vi "Scanner Message Loop.vi"(8 "error in (no error)":errorcluster) -> (0 "error out":errorcluster)   [LabVIEW 2020, in "Hiden Scanner.lvlib"]
doc: "Message loop for handling messages pertaining to the acquisition of data from the hardware."
uses:
  Hiden Scanner.lvlib
  support/PCT FGV CMD.ctl
  Acquisition State.ctl
  Scanner Hardware Configuration.ctl
  support/Message Queue/Message Cluster.ctl
  support/Message Queue/Enqueue Message (Single).vi
  <vilib>/Utility/error.llb/Error Cluster From Error Code.vi
  <vilib>/ErrorRing/Error Ring.xnode
  support/Message Queue/Message Queue.lvlib
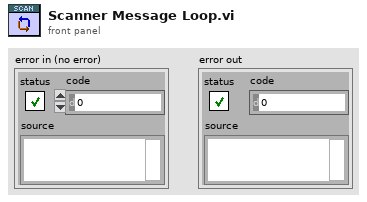
[diagram p1: front panel]
types:
  T1 = typedef "PCT FGV CMD.ctl" = enum16{"INIT", "GET", "SET"}
  T2 = typedef "Message Queue.lvlib/All Message Queues.ctl" = cluster{"UI":refnum<queue>, "Logging":refnum<queue>, "LOG":refnum<queue>, "ALARM":refnum<queue>, "Test":refnum<queue>, "Answer":refnum<queue>, "PLC":refnum<queue>, "DB":refnum<queue>, "Report":refnum<queue>, "OPC":refnum<queue>, "Procedure":refnum<queue>, "PalmSens":refnum<queue>, "SYS 7000 Reader":refnum<queue>, "SWITCH":refnum<queue>, "MOTOR":refnum<queue>, "MOTION":refnum<queue>, "HIDEN":refnum<queue>, "VALVE":refnum<queue>, "MFC":refnum<queue>, "PUMP IN":refnum<queue>, "PUMP OUT":refnum<queue>}
  T3 = typedef "PCT Data REFs.ctl" = cluster{"PLC AI Notifier":refnum<notifier>, "PS Data Queue":refnum<queue>, "BTN Queue":refnum<queue>, "PLC DI notifier":refnum<notifier>, "Timer notifier":refnum<notifier>, "DMM PS":refnum<notifier>, "DMM Gages":refnum<notifier>, "XYZ notifier":refnum<notifier>, "Test Notifier":refnum<notifier>, "Scanner notifier":refnum<notifier>, "OPC Notifier":refnum<notifier>, "HIDEN queue":refnum<queue>}
  T4 = typedef "Hiden Scanner.lvlib/Scanner Hardware Configuration.ctl" = cluster{"Link":cluster{"Connection":enum16{"Serial", "TCP/IP", "USB"}, "Host or IP address (TCP/IP)":string, "Port (Serial/USB)":string}, "VISA resource":refnum<visa-resource-name>, "Writer Queue":refnum<queue>, "Status":bool}
  T5 = typedef "Message Queue.lvlib/Message Cluster.ctl" = cluster{"Message":string, "Message Data":variant}
  T6 = typedef "Hiden Scanner.lvlib/Acquisition State.ctl" = enum16{"Idle", "Initialized"}
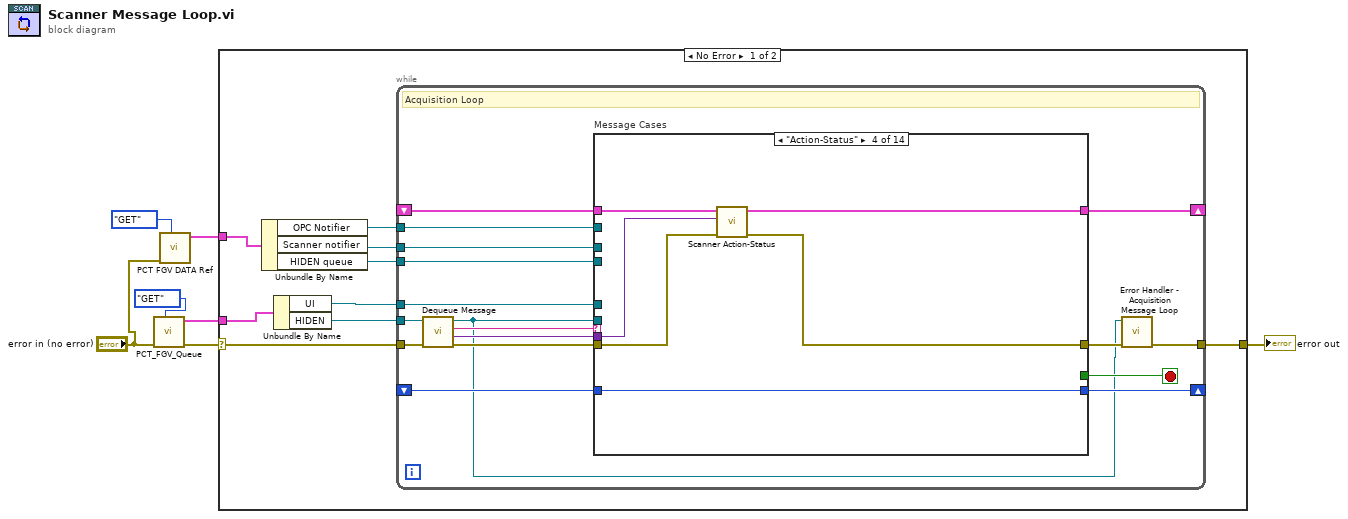
[diagram p0: block diagram]
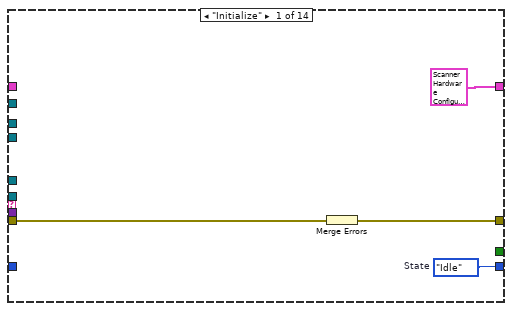
[diagram p2: hidden frame]
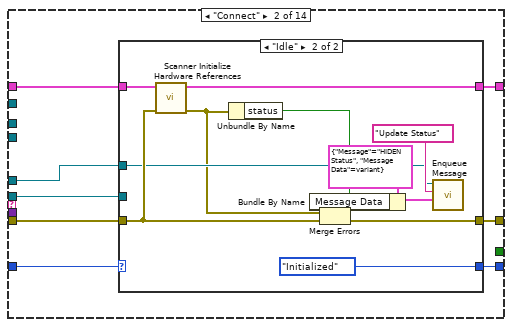
[diagram p3: hidden frame]
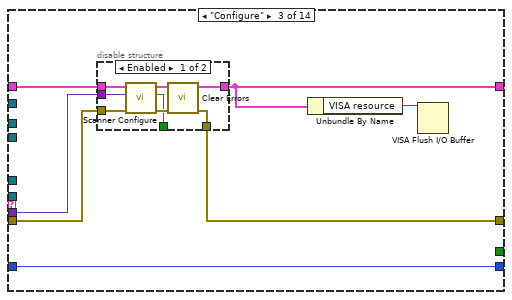
[diagram p5: hidden frame]
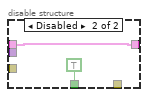
[diagram p6: hidden frame]
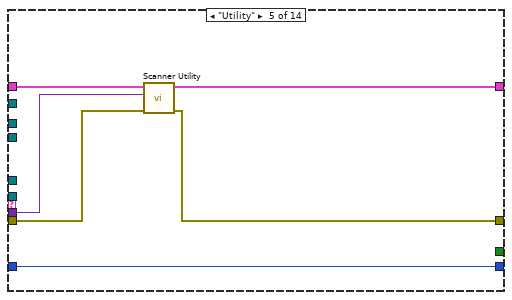
[diagram p7: hidden frame]
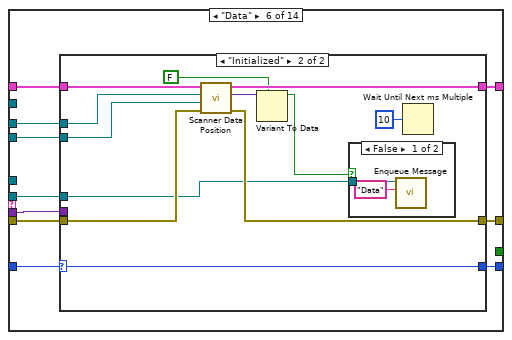
[diagram p8: hidden frame]
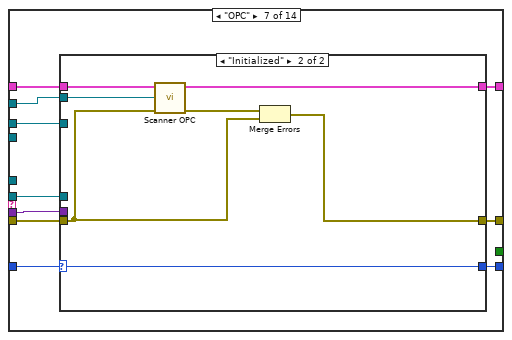
[diagram p11: hidden frame]
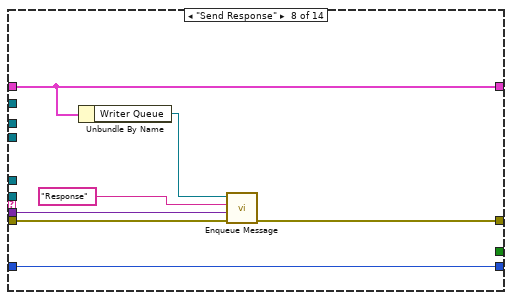
[diagram p13: hidden frame]
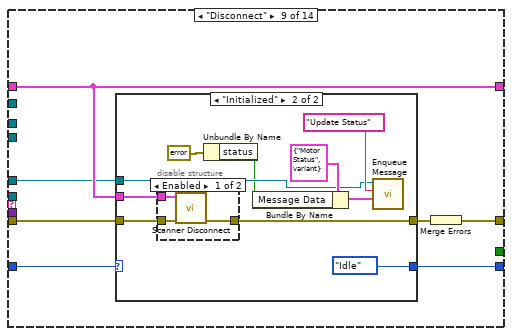
[diagram p14: hidden frame]
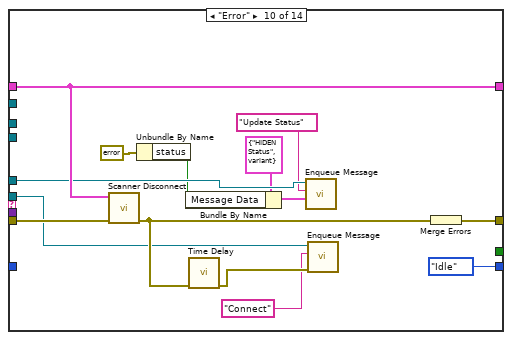
[diagram p17: hidden frame]
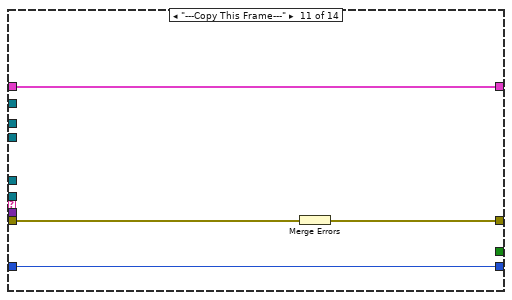
[diagram p18: hidden frame]
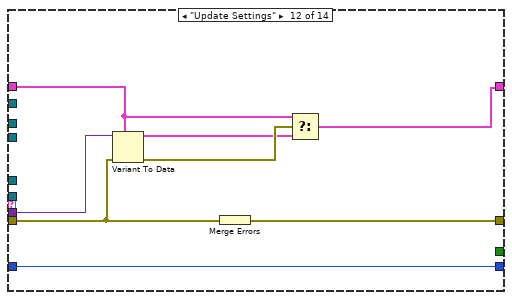
[diagram p19: hidden frame]
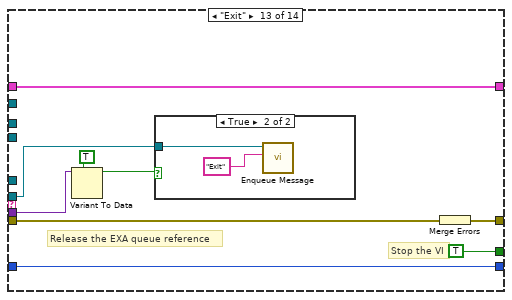
[diagram p20: hidden frame]
diagram:
  n1 = call "PCT_FGV_Queue.vi"("CMD"=PCT_FGV_CMD."GET", "error in (no error)"="error in (no error)") -> ("error out"=w5:errorcluster, "Message Queues out"=w4:T2)  [unwired: 8 in]
  n2 = call "PCT FGV DATA Ref.vi"("CMD"=PCT_FGV_CMD."GET", "error in (no error)"="error in (no error)") -> ("Data REF"=w1:T3)  [unwired: 8 in, 1 out]
  n3 = case shown="No Error" w5 {
    selector: w5 -> [w13 w212]
    tunnel: w4 -> [w16 _]
    tunnel: [w14 w212] -> w7
    tunnel: w1 -> [w11 _]
    frame No Error {
      n4 = Unbundle By Name(w11) -> ("OPC Notifier"=w9:refnum<notifier>, "Scanner notifier"=w10:refnum<notifier>, "HIDEN queue"=w8:refnum<queue>)
      n5 = Unbundle By Name(w16) -> ("UI"=w12:refnum<queue>, "HIDEN"=w15:refnum<queue>)
      n6 = while {
        tunnel: w15 -> [w27]
        shift-right: [w32] -> _
        shift-left: _ -> [w33]
        tunnel: w12 -> [w22]
        shift-right: [w25] -> _
        shift-left: _ -> [w26]
        tunnel: w13 -> [w30]
        tunnel: [w24] -> w14
        tunnel: w10 -> [w20]
        tunnel: w9 -> [w19]
        tunnel: w8 -> [w17]
        stop <- w31 stop-if-true
        # "Acquisition Loop"
        n7 = call "Dequeue Message.vi"("error in (no error)"=w30, "Message Queue"=w27) -> ("error out"=w29:errorcluster, "Message Data"=w28:variant, "Message"=w21:string, "dup Message Queue"=w18:refnum<queue>)  [unwired: 6 in]
        n8 = case "Message Cases" shown="\"Action-Status\"" w21 {
          selector: w21 -> [_ _ _ _ _ _ _ _ _ _ _ _ _ w201]
          tunnel: w18 -> [_ w42 _ _ _ w96 w123 _ _ w165 _ _ w192 _]
          tunnel: w29 -> [w36 w43 w63 w77 w84 w95 w122 w139 w147 w176 w181 w183 w191 _]
          tunnel: [w37 w45 w62 w76 w82 w97 w124 w138 w148 w177 w179 w189 w197 w202] -> w23
          tunnel: w33 -> [_ w44 w64 w78 w86 w93 w120 w136 w145 w175 w180 w185 w196 w204]
          tunnel: [T4 {"Link"={"Connection"=enum."Serial", "Host or IP address (TCP/IP)"="", "Port (Serial/USB)"="COM1"}, "VISA resource"="", "Writer Queue"=refnum, "Status"=FALSE} ("Data Cluster") w41 w61 w79 w83 w94 w121 w136 w145 w175 w180 w184 w196 w204] -> w32
          tunnel: [_ _ _ _ _ _ _ _ _ _ _ _ TRUE _] -> w31
          tunnel: w28 -> [_ _ w65 w80 w85 w90 w117 w137 _ _ _ w188 w190 _]
          tunnel: w22 -> [_ w38 _ _ _ _ _ _ w142 w173 _ _ _ _]
          tunnel: w26 -> [_ w39 w66 w81 w87 w91 w118 w140 w144 _ w178 w182 w195 w203]
          tunnel: [w35 w40 w66 w81 w87 w92 w119 w140 w143 Acquisition_State."Idle" ("State") w178 w182 w195 w203] -> w25
          tunnel: w20 -> [_ _ _ _ _ w89 w116 _ _ _ _ _ _ _]
          tunnel: w19 -> [_ _ _ _ _ _ w115 _ _ _ _ _ _ _]
          tunnel: w17 -> [_ _ _ _ _ w88 _ _ _ _ _ _ _ _]
          frame "Initialize" {
            w35 = Acquisition_State."Idle"  # State
            # "Initialize  - Initialize is currently a no-op.  The hardware initialization takes place in the 'Start' message."
            n9 = Merge Errors(w36) -> (w37:errorcluster)
          }
          frame "Connect" {
            # "Start - Configure and start the acquisition."
            n10 = case shown="\"Idle\"" w39 {
              selector: w39 -> [w46 _]
              tunnel: [w47 w59] -> w45
              tunnel: w44 -> [w48 w58]
              tunnel: w43 -> [w47 w55]
              tunnel: w42 -> [_ _]
              tunnel: [w48 w57] -> w41
              tunnel: [w46 Acquisition_State."Initialized" ("Acquisition State")] -> w40
              tunnel: w38 -> [_ w51]
              frame "Initialized" {
                # "The system is already acquiring. Ignore the \"Start\" message."
              }
              frame "Idle" {
                # "If the system is idle, start the acquisition."
                n11 = call "Scanner Initialize Hardware References.vi"("error in (no error)"=w55, "Hardware Resources in"=w58) -> ("error out"=w49:errorcluster, "Hardware Resources out"=w57:T4)  [unwired: 8 in]
                n12 = Unbundle By Name(w49) -> ("status"=w50:bool)
                n13 = Bundle By Name(cluster=T5 {"Message"="HIDEN Status", "Message Data"=variant} ("Message Cluster"), "Message Data"=w50) -> (w53:T5)
                n14 = Merge Errors(w49, w55) -> (w59:errorcluster)
                n15 = call-poly "Enqueue Message.vi"("Message Data"=w53, "Message"="Update Status", "Message Queue"=w51) -> ()  [unwired: 7 in, 2 out]
              }
            }
          }
          frame "Configure" {
            # "Start - Configure and start the acquisition."
            n16 = disable-structure shown="Enabled" {
              disable-tunnel: w65 -> [w73 _]
              disable-tunnel: w64 -> [w72 w75]
              disable-tunnel: w63 -> [w71 _]
              disable-tunnel: [w69 w75] -> w61
              disable-tunnel: [w68 _] -> w62
              disable-tunnel: [w67 TRUE ("Send Resp")] -> _
              frame Enabled {
                n17 = call "Scanner Configure.vi"("error in (no error)"=w71, "Message Data"=w73, "Data Cluster"=w72) -> ("error out"=w70:errorcluster, "Send Resp"=w67:bool, "Data Cluster out"=w69:T4)  [unwired: 6 in]
                n18 = call <vilib>:"Clear Errors.vi"("error in (no error)"=w70) -> ("error out"=w68:errorcluster)  [unwired: 5 in, 1 out]
              }
              frame Disabled {
              }
            }
            n19 = Unbundle By Name(w61) -> ("VISA resource"=w60:refnum<visa-resource-name>)
            n20 = VISA Flush I/O Buffer(VISA resource name=w60) -> ()  [unwired: 2 in, 2 out]
          }
          frame "Action-Status" {
            # "Start - Configure and start the acquisition."
            n21 = call "Scanner Action-Status.vi"("error in (no error)"=w77, "Message Data"=w80, "Data Cluster"=w78) -> ("error out"=w76:errorcluster, "Data Cluster out"=w79:T4)  [unwired: 7 in]
          }
          frame "Utility" {
            # "Start - Configure and start the acquisition."
            n22 = call "Scanner Utility.vi"("error in (no error)"=w84, "Message Data"=w85, "Data Cluster"=w86) -> ("error out"=w82:errorcluster, "Data Cluster out"=w83:T4)  [unwired: 7 in]
          }
          frame "Data" {
            # "Acquire - Acquire data from the hardware. Since this is a continuous acquisition, this message will always message itself to run again."
            n23 = case shown="\"Initialized\"" w91 {
              selector: w91 -> [w98 w112]
              tunnel: [w99 w109] -> w97
              tunnel: w96 -> [_ w106]
              tunnel: w95 -> [w99 w108]
              tunnel: [w100 w110] -> w94
              tunnel: w93 -> [w100 w111]
              tunnel: [w98 w112] -> w92
              tunnel: w90 -> [_ _]
              tunnel: w89 -> [_ w107]
              tunnel: w88 -> [_ w101]
              frame "Idle" {
              }
              frame "Initialized" {
                # "Read  data"
                n24 = call "Scanner Data Position.vi"("error in (no error)"=w108, "queue"=w101, "Scanner notifier"=w107, "Hardware Resources in"=w111) -> ("error out"=w109:errorcluster, "Message Data Out"=w104:variant, "Hardware Resources out"=w110:T4)  [unwired: 5 in]
                n25 = Variant To Data(type=FALSE, Variant=w104) -> (data=w102:bool)  [unwired: 1 in, 1 out]
                n26 = case shown="False" w102 {
                  tunnel: w106 -> [w114 _]
                  frame False {
                    n27 = call-poly "Enqueue Message.vi"("Message"="Data", "Message Queue"=w114) -> ()  [unwired: 8 in, 2 out]
                  }
                  frame True {
                  }
                }
                n28 = Wait Until Next ms Multiple(millisecond multiple=u32 10) -> ()  [unwired: 1 out]
              }
            }
          }
          frame "OPC" {
            # "Acquire - Acquire data from the hardware. Since this is a continuous acquisition, this message will always message itself to run again."
            n29 = case shown="\"Initialized\"" w118 {
              selector: w118 -> [w125 w133]
              tunnel: [w126 w134] -> w124
              tunnel: w123 -> [_ _]
              tunnel: w122 -> [w126 w130]
              tunnel: [w127 w131] -> w121
              tunnel: w120 -> [w127 w132]
              tunnel: [w125 w133] -> w119
              tunnel: w117 -> [_ _]
              tunnel: w116 -> [_ _]
              tunnel: w115 -> [_ w128]
              frame "Idle" {
              }
              frame "Initialized" {
                # "Read  data"
                n30 = call "Scanner OPC.vi"("error in (no error)"=w130, "OPC Notifier"=w128, "Hardware Resources in"=w132) -> ("error out"=w129:errorcluster, "Hardware Resources out"=w131:T4)  [unwired: 7 in]
                n31 = Merge Errors(w129, w130) -> (w134:errorcluster)
              }
            }
          }
          frame "Send Response" {
            # "Acquire - Acquire data from the hardware. Since this is a continuous acquisition, this message will always message itself to run again."
            n32 = Unbundle By Name(w136) -> ("Writer Queue"=w135:refnum<queue>)
            n33 = call-poly "Enqueue Message.vi"("error in (no error)"=w139, "Message Data"=w137, "Message"="Response", "Message Queue"=w135) -> ("error out"=w138:errorcluster)  [unwired: 6 in, 1 out]
          }
          frame "Disconnect" {
            # "Stop - Stop the Acquisition."
            n34 = case shown="\"Initialized\"" w144 {
              selector: w144 -> [w149 _]
              tunnel: w147 -> [w150 w160]
              tunnel: [w150 w159] -> w146
              tunnel: w145 -> [_ w158]
              tunnel: [w149 Acquisition_State."Idle" ("State")] -> w143
              tunnel: w142 -> [_ w152]
              frame "Idle" {
                # "The system is already idle. Ignore the \"Stop\" message."
              }
              frame "Initialized" {
                # "If the system is acquiring, stop the acquisition."
                n35 = disable-structure shown="Enabled" {
                  disable-tunnel: w160 -> [w163 _]
                  disable-tunnel: [w162 _] -> w159
                  disable-tunnel: w158 -> [w161 _]
                  frame Enabled {
                    n36 = call "Scanner Disconnect.vi"("error in (no error)"=w163, "Hardware Resources in"=w161) -> ("error out"=w162:errorcluster)  [unwired: 9 in]
                  }
                  frame Disabled {
                  }
                }
                n37 = Unbundle By Name(errorcluster {"status"=TRUE, "code"=6001, "source"=""} ("error out")) -> ("status"=w151:bool)
                n38 = Bundle By Name(cluster=T5 {"Message"="Motor Status", "Message Data"=variant} ("Message Cluster"), "Message Data"=w151) -> (w155:T5)
                n39 = call-poly "Enqueue Message.vi"("Message Data"=w155, "Message"="Update Status", "Message Queue"=w152) -> ()  [unwired: 7 in, 2 out]
              }
            }
            n40 = Merge Errors(w146) -> (w148:errorcluster)
          }
          frame "Error" {
            # "Stop - Stop the Acquisition."
            n41 = call "Scanner Disconnect.vi"("error in (no error)"=w176, "Hardware Resources in"=w175) -> ("error out"=w167:errorcluster)  [unwired: 9 in]
            n42 = Unbundle By Name(errorcluster {"status"=TRUE, "code"=6001, "source"=""} ("error out")) -> ("status"=w168:bool)
            n43 = Bundle By Name(cluster=T5 {"Message"="HIDEN Status", "Message Data"=variant} ("Message Cluster"), "Message Data"=w168) -> (w171:T5)
            n44 = call "Time Delay"("error in (no error)"=w167) -> ("error out"=w166:errorcluster)  [unwired: 10 in]
            n45 = call-poly "Enqueue Message.vi"("Message Data"=w171, "Message"="Update Status", "Message Queue"=w173) -> ()  [unwired: 7 in, 2 out]
            n46 = call-poly "Enqueue Message.vi"("error in (no error)"=w166, "Message"="Connect", "Message Queue"=w165) -> ()  [unwired: 7 in, 2 out]
            n47 = Merge Errors(w167) -> (w177:errorcluster)
          }
          frame "---Copy This Frame---" {
            # "Duplicate this frame when creating new messages.  Change this comment in the duplicated frame to describe this message."
            n48 = Merge Errors(w181) -> (w179:errorcluster)
          }
          frame "Update Settings" {
            # "New settings are available, update the current ones stored in the shift register with the settings sent as part of the message"
            n49 = Variant To Data(error in=w183, type=w185, Variant=w188) -> (data=w186:T4, error out=w187:errorcluster)
            n50 = Merge Errors(w183) -> (w189:errorcluster)
            n51 = Select(t=w185, s=w187, f=w186) -> (s? t:f=w184:T4)
          }
          frame "Exit" {
            # "Release the EXA queue reference"
            # "Stop the VI"
            # "Exit - Send the Exit message to the UI Message Handler."
            n52 = Variant To Data(type=TRUE, Variant=w190) -> (data=w194:bool)  [unwired: 1 in, 1 out]
            n53 = case shown="True" w194 {
              tunnel: w192 -> [_ w200]
              frame False {
              }
              frame True {
                n54 = call-poly "Enqueue Message.vi"("Message"="Exit", "Message Queue"=w200) -> ()  [unwired: 8 in, 2 out]
              }
            }
            n55 = Merge Errors(w191) -> (w197:errorcluster)
          }
          frame Default {
            # "'Default' case only runs if there is a message that isn't defined in any of the other cases.  Output a programming error."
            n56 = xnode "Error Ring"("parameter 0"=w201) -> ("error out"=w202:errorcluster)
          }
        }
        n57 = call "Error Handler - Acquisition Message Loop.vi"("error in (no error)"=w23, "Message Queue"=w18) -> ("dup error in"=w24:errorcluster)  [unwired: 8 in, 1 out]
      }
    }
    frame Error {
    }
  }
  "error out" <- w7
